vi "Check file name for validity.vi"(0 "String in":string, 11 "error in (no error)":errorcluster) -> (4 "String out":string, 8 "Valid File of folder name":bool, 15 "error out":errorcluster)   [LabVIEW 2011]
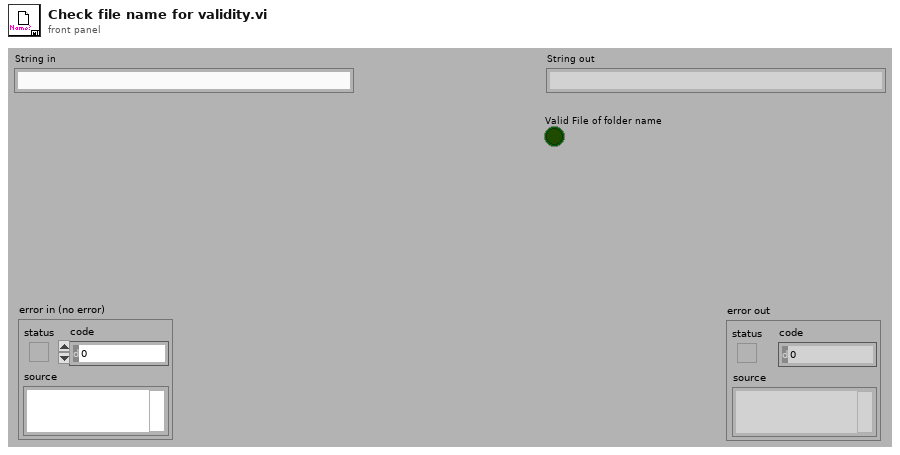
[diagram p1: front panel]
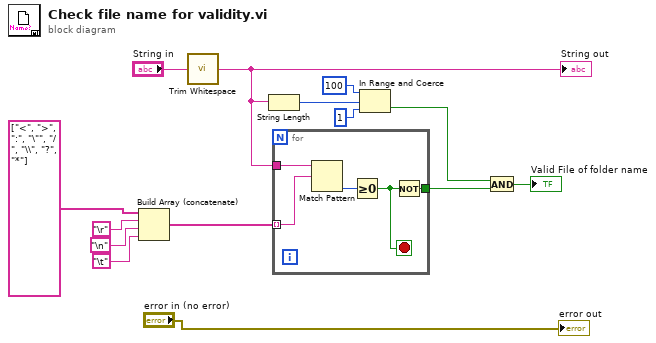
[diagram p0: block diagram]
diagram:
  n1 = Build Array (concatenate)(string[] ["<", ">", ":", "\"", "/", "\\", "?", "*"], "\r", "\n", "\t") -> (w10:string[])
  n2 = call <vilib>:"Trim Whitespace.vi"("string"="String in") -> ("trimmed string"=w2:string)  [unwired: 1 in]
  "String out" <- w2
  n3 = String Length(string=w2) -> (length=w8:i32)
  n4 = for {
    tunnel: w2 -> [w19]
    tunnel: w10 -> [w18] mode=indexing
    tunnel: [w15] -> w7
    stop <- w16 stop-if-true
    n5 = Match Pattern(string=w19, regular expression=w18) -> (offset past match=w17:i32)  [unwired: 1 in, 3 out]
    n6 = Greater Or Equal To 0?(x=w17) -> (x >= 0?=w16:bool)
    n7 = Not(x=w16) -> (.not. x?=w15:bool)
  }
  n8 = In Range and Coerce(upper limit=100, x=w8, lower limit=1) -> (In Range?=w6:bool)  [unwired: 1 out]
  n9 = And(x=w6, y=w7) -> (x .and. y?=→"Valid File of folder name":bool)
  "error out" <- "error in (no error)"
